vi "Manual.vi"(6 "Cluster":T12={"VISA resource name"="", "baud rate "=9600}, 7 "vi reference":refnum<vi>, 8 "error in (no error)":errorcluster, 9 "IOList_280":T1, 11 "Manual":T4(tab)) -> (0 "error out":errorcluster, 3 "Out reference":refnum<vi>)   [LabVIEW 2015]
uses:
  Control Button/Exit.ctl
  Control Button/Scanner config.ctl
  Control Button/Save.ctl
  Galobal variable_TI.vi
  <vilib>/addons/database/Connection.llb/DB Tools Open Connec (String).vi
  <vilib>/Instr/_visa.llb/VISA Configure Serial Port (Instr).vi
  <vilib>/addons/database/_DB Variant To Data/Database Variant To Data.xnode
  <vilib>/addons/database/NI_Database_API.lvlib
panel:
  out "Array":string[](array[string])
  out "Byte Lenth":i32
  out "error out 2":errorcluster
  out "Manual DO":bool[](array[boolean])
  in  "Stop":T2
  out "NewVal":T3
  in  "Digital Output":T5
  out "LVDT":string
  out "Digital Input":T6
  in  "Home Calling M1":bool
  in  "Stop M1":bool
  in  "SERVO ON CMD M1":bool
  in  "Speed (mm/s) M1":i32=10
  in  "Travel (mm)M1":i32=5
  out "STM1 Done Bit":bool
  out "Error Message":string
  out "Load Cell":dbl format="%0.03f"
  in  "Model Trigger":bool
  in  "Program List 2":string(combo)="VW Medium"
  out "Camera Status":T7
  in  "Save":T8
  out "Analog Input":T9 {"Analog Data 6" format="%0.02f"; "Analog Data 5" format="%0.02f"; "Analog Data 4" format="%0.02f"; "Analog Data 3" format="%0.02f"; "Analog Data 2" format="%0.02f"; "Analog Data" format="%0.02f"}
  in  "Sensor Data 3":T10
  out "Error Status":bool
  in  "Scanner config":T11
  out "Read data":string
  out "Boolean":bool
  # "Instruction for Servo motor Operate\n(1)  Switch  ON -OFF  of Fixture Slide servo Brake ON Cmd (P0.19)  \n      from Digital Output tab.\n(2) Switch  ON -OFF  of Fixture Slide Servo Direction Command (P0.20)\n      from Digital Output tab."
  # "Fixture Slide servo"
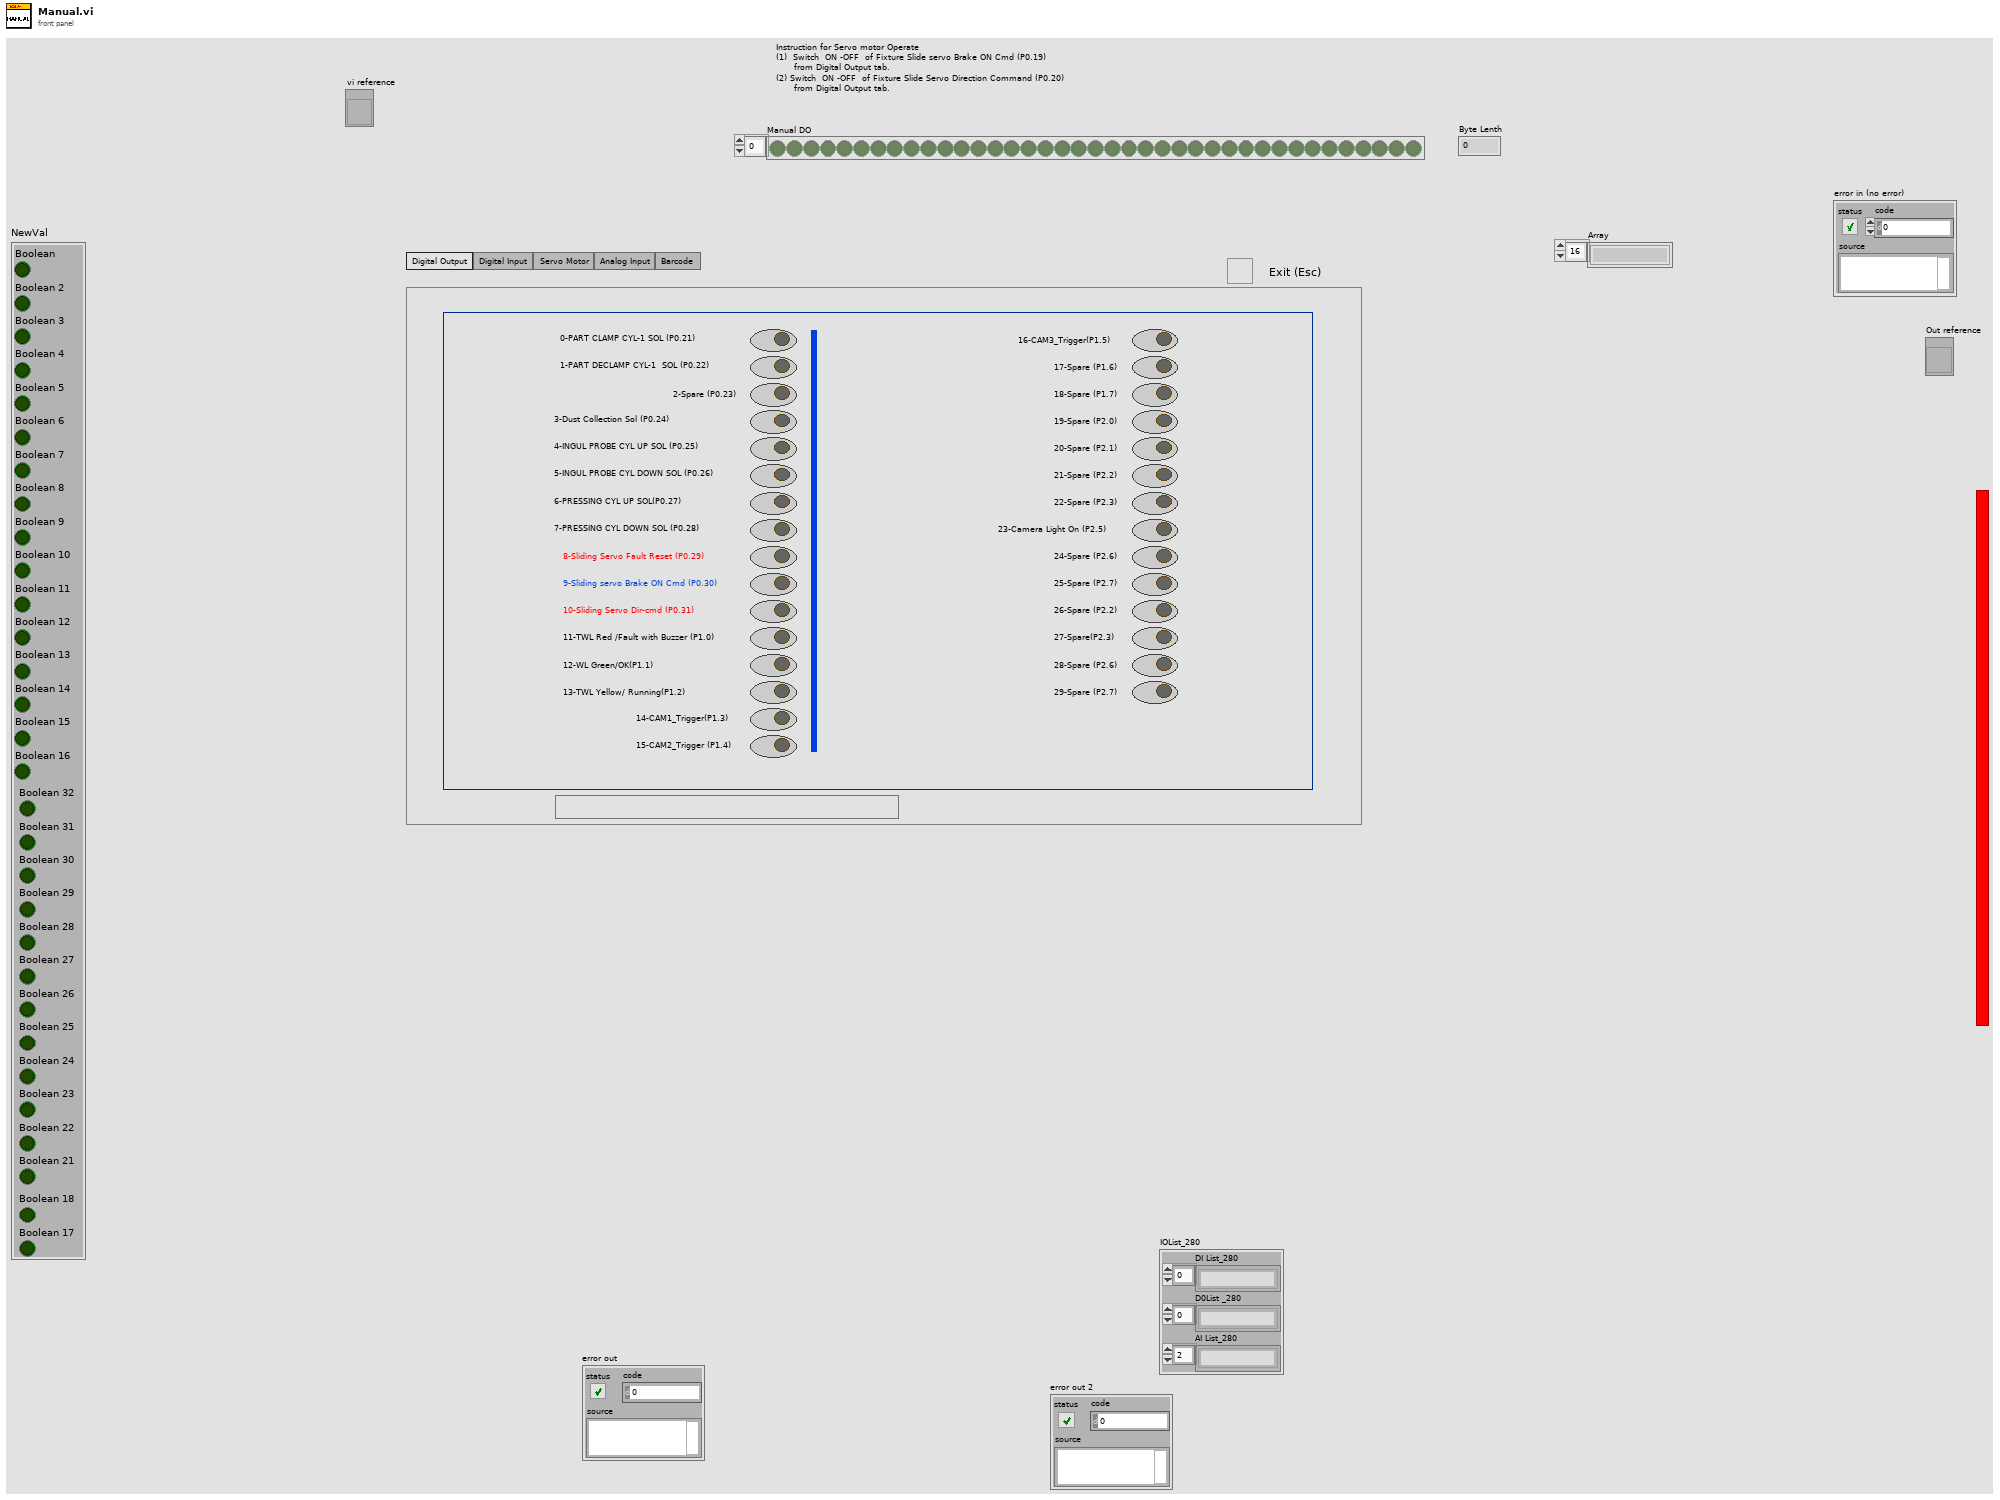
[diagram p1: front panel]
types:
  T1 = cluster{"DI List_280":string[], "D0List _280":string[], "AI List_280":string[]}
  T2 = typedef "Exit.ctl" = bool
  T3 = cluster{"Boolean":bool, "Boolean 2":bool, "Boolean 3":bool, "Boolean 4":bool, "Boolean 5":bool, "Boolean 6":bool, "Boolean 7":bool, "Boolean 8":bool, "Boolean 9":bool, "Boolean 10":bool, "Boolean 11":bool, "Boolean 12":bool, "Boolean 13":bool, "Boolean 14":bool, "Boolean 15":bool, "Boolean 16":bool, "Boolean 17":bool, "Boolean 18":bool, "Boolean 21":bool, "Boolean 22":bool, "Boolean 23":bool, "Boolean 24":bool, "Boolean 25":bool, "Boolean 26":bool, "Boolean 27":bool, "Boolean 28":bool, "Boolean 29":bool, "Boolean 30":bool, "Boolean 31":bool, "Boolean 32":bool}
  T4 = enum32{"Digital Output", "Digital Input", "Servo Motor ", "Analog Input", "Barcode "}
  T5 = cluster{"DO.00":bool, "DO.01":bool, "DO.02":bool, "DO.03":bool, "DO.04":bool, "DO.05":bool, "DO.06":bool, "DO.06":bool, "DO.07":bool, "DO.08":bool, "DO.09":bool, "DO.10":bool, "DO.11":bool, "DO.12":bool, "DO.13":bool, "DO.14":bool, "DO.07 2":bool, "DO.08 2":bool, "DO.09 2":bool, "DO.10 2":bool, "DO.11 2":bool, "DO.12 2":bool, "DO.13 2":bool, "DO.14 2":bool, "DO.00 2":bool, "DO.01 2":bool, "DO.02 2":bool, "DO.03 2":bool, "DO.06 2":bool, "DO.06 3":bool}
  T6 = cluster{"Digital Input":bool, "Digital Input 2":bool, "Digital Input 3":bool, "Digital Input 4":bool, "Digital Input 5":bool, "Digital Input 6":bool, "Digital Input 7":bool, "Digital Input 8":bool, "Digital Input 9":bool, "Digital Input 10":bool, "Digital Input 11":bool, "Digital Input 12":bool, "Digital Input 13":bool, "Digital Input 14":bool, "Digital Input 15":bool, "Digital Input 16":bool, "Digital Input 17":bool, "Digital Input 18":bool, "Digital Input 19":bool, "Digital Input 20":bool, "Digital Input 21":bool, "Digital Input 22":bool, "Digital Input 23":bool, "Digital Input 24":bool, "Digital Input 25":bool, "Digital Input 26":bool, "Digital Input 27":bool, "Digital Input 28":bool, "Digital Input 29":bool, "Digital Input 30":bool, "Digital Input 31":bool, "Digital Input 32":bool, "Digital Input 33":bool, "Digital Input 34":bool, "Digital Input 35":bool, "Digital Input 36":bool, "Digital Input 37":bool, "Digital Input 38":bool, "Digital Input 39":bool, "Digital Input 40":bool, "Digital Input 41":bool, "Digital Input 42":bool, "Digital Input 43":bool, "Digital Input 44":bool, "Digital Input 45":bool, "Digital Input 46":bool, "Digital Input 47":bool, "Digital Input 48":bool, "Digital Input 49":bool, "Digital Input 50":bool, "Digital Input 51":bool}
  T7 = cluster{"Left CAM OK":bool, "Left CAM NG":bool, "Right CAM OK":bool, "Right CAM NG":bool, "LCD  CAM OK":bool, "LCD CAM NG ":bool}
  T8 = typedef "Save.ctl" = bool
  T9 = cluster{"Analog Data":dbl, "Analog Data 2":dbl, "Analog Data 3":dbl, "Analog Data 4":dbl, "Analog Data 5":dbl, "Analog Data 6":dbl, "IL Sensor1_AI6":bool, "IL Sensor1_AI7":bool, "IL Sensor1_AI8":bool, "IL Sensor1_AI9":bool}
  T10 = cluster{"IL Sensor_Max (AI6)":dbl, "IL Sensor_Min (AI6)":dbl, "IL Sensor_Max (AI7)":dbl, "IL Sensor _Min (AI7)":dbl, "IL Sensor_Max (AI8)":dbl, "IL Sensor_Min (AI8)":dbl, "IL Sensor_Max  (AI9)":dbl, "IL Sensor_Min  (AI9)":dbl}
  T11 = typedef "Scanner config.ctl" = bool
  T12 = cluster{"VISA resource name":refnum<visa-resource-name>, "baud rate ":u32}
  T13 = typedef "NI_Database_API.lvlib/Conn ObjectReference.ctl" = refnum<k1>
  T14 = cluster{" Fixture Brack on":refnum<vi>, " Fixture Direction":refnum<vi>, "Servo Cmd":refnum<vi>, "Servo Home":refnum<vi>}
  T15 = cluster{"Digital input[0]":bool, "Digital input[1]":bool, "Digital input[2]":bool, "Digital input[3]":bool, "Digital input[4]":bool, "Digital input[5]":bool, "Digital input[6]":bool, "Digital input[7]":bool, "Digital input[8]":bool, "Digital input[9]":bool, "Digital input[10]":bool, "Digital input[11]":bool, "Digital input[12]":bool, "Digital input[13]":bool, "Digital input[14]":bool, "Digital input[15]":bool, "Digital input[16]":bool, "Digital input[17]":bool, "Digital input[18]":bool, "Digital input[19]":bool, "Digital input[20]":bool, "Digital input[21]":bool, "Digital input[22]":bool, "Digital input[23]":bool, "Digital input[24]":bool, "Digital input[25]":bool, "Digital input[26]":bool, "Digital input[27]":bool, "Digital input[28]":bool, "Digital input[29]":bool, "Digital input[30]":bool, "Digital input[31]":bool, "Digital input[32]":bool, "Digital input[33]":bool, "Digital input[34]":bool, "Digital input[35]":bool, "Digital input[36]":bool, "Digital input[37]":bool, "Digital input[38]":bool, "Digital input[39]":bool, "Digital input[40]":bool, "Digital input[41]":bool, "Digital input[42]":bool, "Digital input[43]":bool, "Digital input[44]":bool, "Digital input[45]":bool, "Digital input[46]":bool, "Digital input[47]":bool, "Digital input[48]":bool, "Digital input[49]":bool, "Digital input[50]":bool}
  T16 = cluster{"Load(AI0) ":dbl, "Load (AI1) ":dbl, "IL Sensor (AI6)":dbl, "IL Sensor  (AI7)":dbl, "IL Sensor (AI8)":dbl, "IL Sensor  (AI9)":dbl, "IL Sensor1_AI6":bool, "IL Sensor1_AI7":bool, "IL Sensor1_AI8":bool, "IL Sensor1_AI9":bool}
  T17 = cluster{"IL Sensor_Max (AI6)":dbl, "IL Sensor_Min (AI6)":dbl, "IL Sensor_Max (AI7)":dbl, "IL Sensor _Min (AI7)":dbl, "IL Sensor_Max (AI8)":dbl, "IL Sensor_Min (AI8)":dbl, "IL Sensor_Max  (AI9)":dbl, "IL Sensor_Min  (AI9)":dbl, "Key":string}
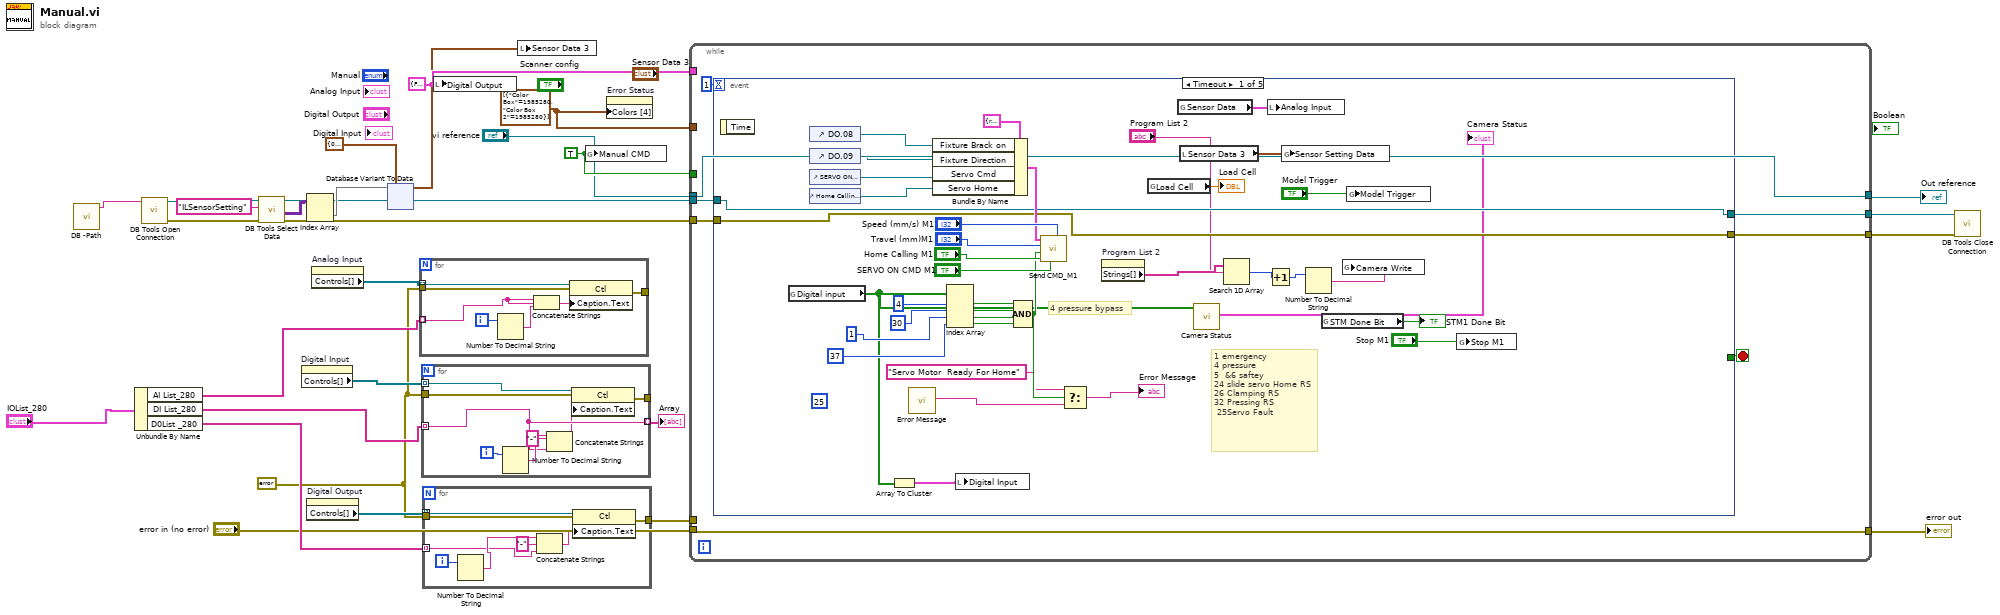
[diagram p0: block diagram]
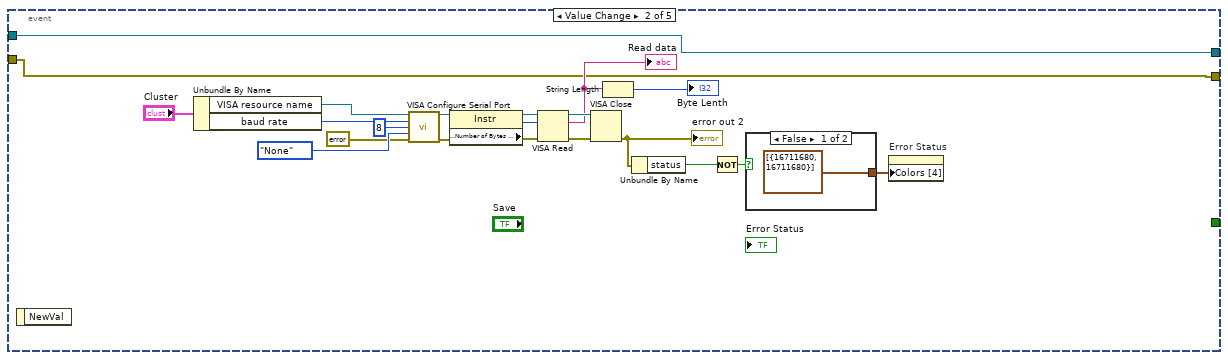
[diagram p2: hidden frame]
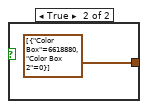
[diagram p3: hidden frame]
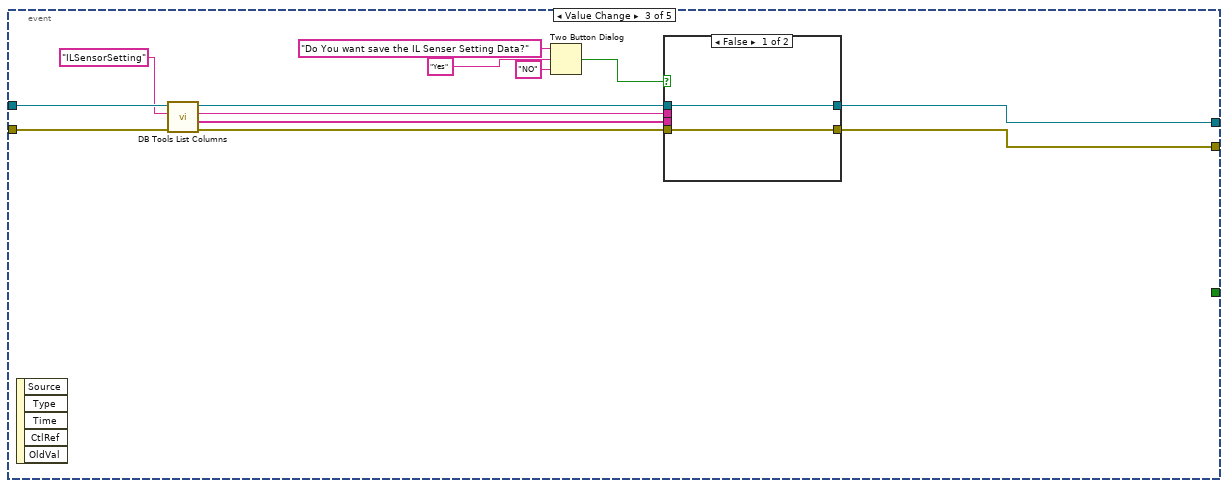
[diagram p4: hidden frame]
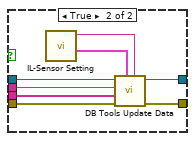
[diagram p5: hidden frame]
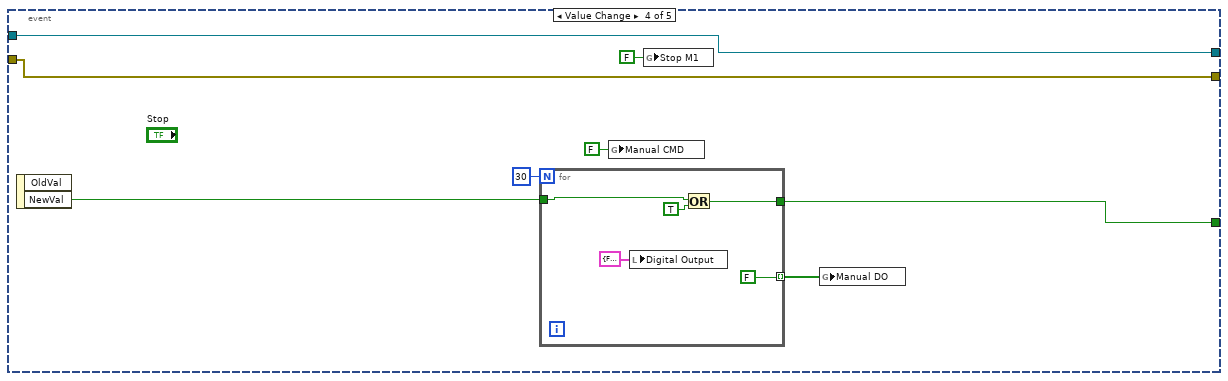
[diagram p6: hidden frame]
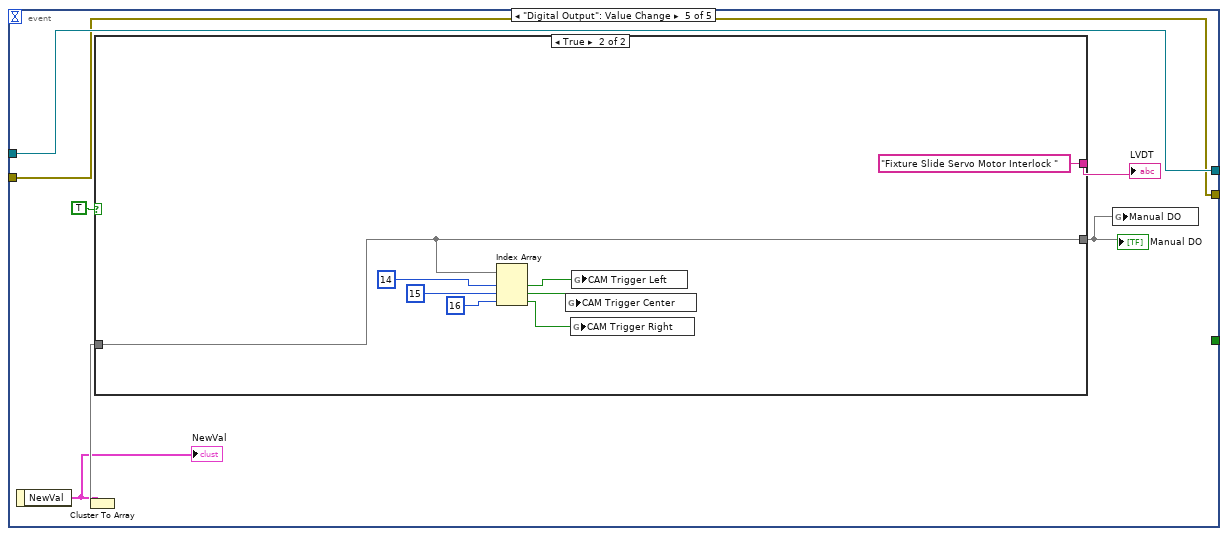
[diagram p7: hidden frame]
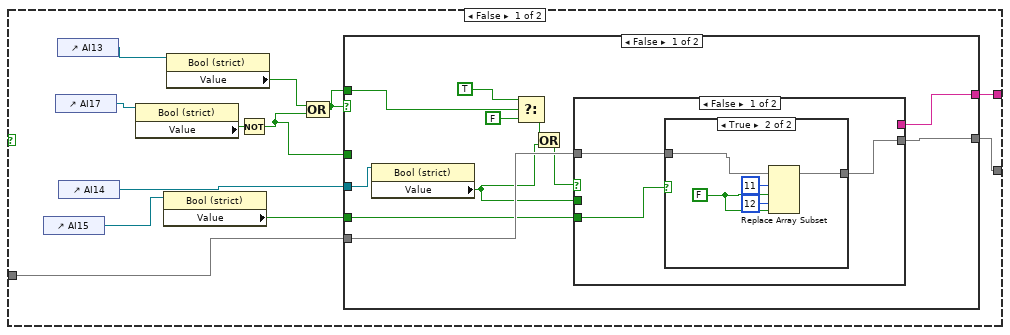
[diagram p8: hidden frame]
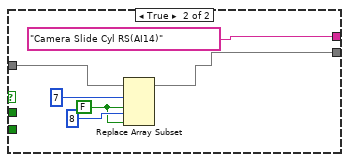
[diagram p10: hidden frame]
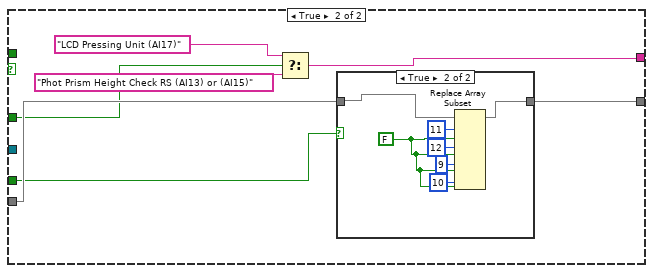
[diagram p11: hidden frame]
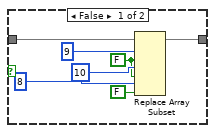
[diagram p12: hidden frame]
diagram:
  w13 = T5 {"DO.00"=FALSE, "DO.01"=FALSE, "DO.02"=FALSE, "DO.03"=FALSE, "DO.04"=FALSE, "DO.05"=FALSE, "DO.06"=FALSE, "DO.06"=FALSE, "DO.07"=FALSE, "DO.08"=FALSE, "DO.09"=FALSE, "DO.10"=FALSE, "DO.11"=FALSE, "DO.12"=FALSE, "DO.13"=FALSE, "DO.14"=FALSE, "DO.07 2"=FALSE, "DO.08 2"=FALSE, "DO.09 2"=FALSE, "DO.10 2"=FALSE, "DO.11 2"=FALSE, "DO.12 2"=FALSE, "DO.13 2"=FALSE, "DO.14 2"=FALSE, "DO.00 2"=FALSE, "DO.01 2"=FALSE, "DO.02 2"=FALSE, "DO.03 2"=FALSE, "DO.06 2"=FALSE, "DO.06 3"=FALSE} ("Digital Output")
  w16 = errorcluster {"status"=FALSE, "code"=0, "source"=""} ("error in (no error)")
  w19 = cluster{"Color Box":u32, "Color Box 2":u32}[] [{"Color Box"=1985280, "Color Box 2"=1985280}] ("Colors [4]")
  w25 = TRUE ("Manual CMD")
  n1 = call "DB -Path.vi"() -> ("String"=w8:string)  [unwired: 11 in]
  n2 = Unbundle By Name("IOList_280") -> ("AI List_280"=w20:string[], "DI List_280"=w22:string[], "D0List _280"=w24:string[])
  n3 = call-poly <vilib>:"DB Tools Open Connection.vi"("connection information"=w8) -> ("error out"=w6:errorcluster, "connection reference"=w7:T13)  [unwired: 7 in]
  n4 = call <vilib>:"DB Tools Select Data.vi"("error in (no error)"=w6, "table"="ILSensorSetting", "connection reference"=w7) -> ("error out"=w4:errorcluster, "data"=w9:variant[][], "connection reference out"=w5:T13)  [unwired: 3 in]
  n5 = property on="Digital Input" class="Clust (strict)"() -> ("Controls[]"=w23:refnum<vi>[])  [unwired: 2 in, 2 out]
  n6 = Index Array(array=w9) -> (element=w10:variant[])  [unwired: 2 in]
  n7 = property on="Digital Output" class="Clust (strict)"() -> ("Controls[]"=w28:refnum<vi>[])  [unwired: 2 in, 2 out]
  n8 = property on="Analog Input" class="Clust (strict)"() -> ("Controls[]"=w21:refnum<vi>[])  [unwired: 2 in, 2 out]
  n9 = xnode "Database Variant To Data"("database variant"=w10, "type"=T10 {"IL Sensor_Max (AI6)"=0.0, "IL Sensor_Min (AI6)"=0.0, "IL Sensor_Max (AI7)"=0.0, "IL Sensor _Min (AI7)"=0.0, "IL Sensor_Max (AI8)"=0.0, "IL Sensor_Min (AI8)"=0.0, "IL Sensor_Max  (AI9)"=0.0, "IL Sensor_Min  (AI9)"=0.0} ("Sensor Setting Data")) -> ("data"=w1:T10)  [unwired: 1 in, 1 out]
  n10 = for {
    tunnel: w21 -> [w35] mode=indexing
    tunnel: [w33] -> _
    tunnel: w16 -> [w31]
    tunnel: w20 -> [w30] mode=indexing
    i -> [w34]
    n11 = Number To Decimal String(number=w34) -> (decimal integer string=w32:string)  [unwired: 1 in]
    n12 = Concatenate Strings(w30, w32) -> ()  [unwired: 1 out]
    n13 = property class="Ctl"(reference=w35, error in=w31, "Caption.Text"=w30) -> (error out=w33:errorcluster)  [unwired: 1 out]
  }
  n14 = for {
    tunnel: w23 -> [w43] mode=indexing
    tunnel: [w41] -> _
    tunnel: w16 -> [w40]
    tunnel: w22 -> [w37] mode=indexing
    tunnel: [w37] -> w17 mode=indexing
    i -> [w42]
    n15 = Number To Decimal String(number=w42) -> (decimal integer string=w39:string)  [unwired: 1 in]
    n16 = Concatenate Strings(w39, "-" ("string"), w37) -> (w36:string)
    n17 = property class="Ctl"(reference=w43, error in=w40, "Caption.Text"=w36) -> (error out=w41:errorcluster)  [unwired: 1 out]
  }
  "Array" <- w17
  n18 = for {
    tunnel: w28 -> [w51] mode=indexing
    tunnel: [w49] -> w29
    tunnel: w16 -> [w48]
    tunnel: w24 -> [w44] mode=indexing
    i -> [w50]
    n19 = Number To Decimal String(number=w50) -> (decimal integer string=w45:string)  [unwired: 1 in]
    n20 = Concatenate Strings(w45, "-" ("string"), w44) -> (w47:string)
    n21 = property class="Ctl"(reference=w51, error in=w48, "Caption.Text"=w47) -> (error out=w49:errorcluster)  [unwired: 1 out]
  }
  n22 = local write "Digital Output"(w13) -> ()
  n23 = local write "Sensor Data 3"(w1) -> ()
  n24 = global write "Galobal variable_TI.vi" "Manual CMD"(w25) -> ()
  n25 = property on="Error Status" class="Bool (strict)"("Colors [4]"=w19) -> ()  [unwired: 2 in, 2 out]
  n26 = while {
    tunnel: w29 -> [_]
    tunnel: [w57] -> w27
    tunnel: "vi reference" -> [w58]
    tunnel: [w58] -> w26
    tunnel: w25 -> [_]
    tunnel: w19 -> [_]
    tunnel: "error in (no error)" -> [w57]
    tunnel: w13 -> [_]
    tunnel: w5 -> [w55]
    tunnel: w4 -> [w54]
    tunnel: [w53] -> w3
    tunnel: [w52] -> w2
    stop <- w56 stop-if-true
    n27 = event shown="[0] Timeout" {
      selector: _ -> [_ _ _ _ _]
      dyn-events: _ -> [_ _ _ _ _]
      timeout: 1 -> [_ _ _ _ _]
      tunnel: [_ _ _ w145 _] -> w56
      tunnel: w55 -> [w71 w99 w132 w144 w157]
      tunnel: w54 -> [w70 w98 w131 w143 w156]
      tunnel: [w71 w99 w126 w144 w157] -> w53
      tunnel: [w70 w98 w125 w143 w156] -> w52
      event Timeout {
        (unwired) 25 ("index")
        # "4 pressure bypass"
        # "1 emergency\n4 pressure\n5  &6 saftey\n24 slide servo Home RS\n26 Clamping RS\n32 Pressing RS \n 25Servo Fault"
        n28 = event-data() -> ()  [unwired: 1 in, 1 out]
        n29 = global read "Galobal variable_TI.vi" "Digital input"() -> (w61:bool[])
        n30 = control-ref of="DO.08"() -> (w75:refnum<vi>)
        n31 = control-ref of="DO.09"() -> (w74:refnum<vi>)
        n32 = control-ref of="SERVO ON CMD M1"() -> (w89:refnum<vi>)
        n33 = control-ref of="Home Calling M1"() -> (w90:refnum<vi>)
        n34 = Array To Cluster(array=w61) -> (cluster=w97:T15)
        n35 = call "Error Message.vi"() -> ("Error"=w80:string)  [unwired: 11 in]
        n36 = Bundle By Name(cluster=T14 {" Fixture Brack on"=refnum, " Fixture Direction"=refnum, "Servo Cmd"=refnum, "Servo Home"=refnum} ("Slide Servo"), "Fixture Brack on"=w75, "Fixture Direction"=w74, "Servo Cmd"=w89, "Servo Home"=w90) -> (w88:T14)
        n37 = Index Array(array=w61, index #1=4 ("index"), index #2=30 ("index"), index #3=1 ("index"), index #4=37 ("index")) -> (element #1=w84:bool, element #2=w76:bool, element #3=w69:bool, element #4=w78:bool)
        n38 = local write "Digital Input"(w97) -> ()
        n39 = Compound Arithmetic op=AND(w84, w76, w69, w78) -> (w82:bool)
        n40 = call "Send CMD_M1.vi"("Speed (mm/s) M1"="Speed (mm/s) M1", "SERVO ON CMD M1"="SERVO ON CMD M1", "Home Calling M1"="Home Calling M1", "Pokayoka"=w82, "Travel (mm)M1"="Travel (mm)M1", "Slide Servo"=w88) -> ()  [unwired: 6 in]
        n41 = Select(t="Servo Motor  Ready For Home", s=w82, f=w80) -> (s? t:f=→"Error Message":string)
        n42 = property on="Program List 2" class="CmbBox"() -> ("Strings[]"=w63:string[])  [unwired: 2 in, 2 out]
        n43 = global read "Galobal variable_TI.vi" "Load Cell"() -> (→"Load Cell":dbl)
        n44 = global read "Galobal variable_TI.vi" "Sensor Data"() -> (w73:T16)
        n45 = local read "Sensor Data 3"() -> (w72:T10)
        n46 = call "Camera Status.vi"("Digital input"=w61) -> ("Camera Status"=→"Camera Status":T7)  [unwired: 10 in]
        n47 = Search 1D Array(1D array=w63, element="Program List 2") -> (index of element=w65:i32)  [unwired: 1 in]
        n48 = local write "Analog Input"(w73) -> ()
        n49 = Increment(x=w65) -> (x+1=w66:i32)
        n50 = global write "Galobal variable_TI.vi" "Sensor Setting Data"(w72) -> ()
        n51 = Number To Decimal String(number=w66) -> (decimal integer string=w67:string)  [unwired: 1 in]
        n52 = global read "Galobal variable_TI.vi" "STM Done Bit"() -> (→"STM1 Done Bit":bool)
        n53 = global write "Galobal variable_TI.vi" "Camera Write"(w67) -> ()
        n54 = global write "Galobal variable_TI.vi" "Model Trigger"("Model Trigger") -> ()
        n55 = global write "Galobal variable_TI.vi" "Stop M1"("Stop M1") -> ()
      }
      event Value Change {
        n56 = event-data() -> ()  [unwired: 1 in, 1 out]
        n57 = Unbundle By Name("Cluster") -> ("VISA resource name"=w118:refnum<visa-resource-name>, "baud rate"=w117:u32)
        n58 = call-poly "VISA Configure Serial Port"("VISA resource name"=w118, "baud rate (9600)"=w117, "data bits (8)"=u16 8, "parity (0:none)"=enum16{"None", "Odd", "Even", "Mark", "Space"}."None", "error in (no error)"=errorcluster {"status"=FALSE, "code"=0, "source"=""} ("error in (no error) 2")) -> ("VISA resource name out"=w116:refnum<visa-resource-name>, "error out"=w114:errorcluster)  [unwired: 9 in]
        n59 = property class="Instr"(reference=w116, error in=w114) -> (reference out=w115:refnum<visa-resource-name>, error out=w113:errorcluster, "Serial Settings:Number of Bytes at Serial Port"=w112:u32)
        n60 = VISA Read(VISA resource name=w115, byte count=w112, error in (no error)=w113) -> (VISA resource name out=w110:refnum<visa-resource-name>, read buffer=w108:string, error out=w109:errorcluster)  [unwired: 1 out]
        "Read data" <- w108
        n61 = VISA Close(VISA resource name=w110, error in (no error)=w109) -> (error out=w106:errorcluster)
        "error out 2" <- w106
        n62 = String Length(string=w108) -> (length=→"Byte Lenth":i32)
        n63 = Unbundle By Name(w106) -> ("status"=w105:bool)
        n64 = Not(x=w105) -> (.not. x?=w103:bool)
        n65 = case shown="False" w103 {
          tunnel: [cluster{"Color Box":u32, "Color Box 2":u32}[] [{"Color Box"=16711680, "Color Box 2"=16711680}] ("Colors [4]") cluster{"Color Box":u32, "Color Box 2":u32}[] [{"Color Box"=6618880, "Color Box 2"=0}] ("Colors [4]")] -> w104
          frame False {
          }
          frame True {
          }
        }
        n66 = property on="Error Status" class="Bool (strict)"("Colors [4]"=w104) -> ()  [unwired: 2 in, 2 out]
      }
      event Value Change {
        w128 = "ILSensorSetting" ("table")
        n67 = event-data() -> ()  [unwired: 1 in, 5 out]
        n68 = call <vilib>:"DB Tools List Columns.vi"("error in (no error)"=w131, "table"=w128, "connection reference"=w132) -> ("error out"=w129:errorcluster, "columns"=w127:string[], "connection reference out"=w130:T13)  [unwired: 1 in, 1 out]
        n69 = Two Button Dialog(message="Do You want save the IL Senser Setting Data?", 1:"NO" ("F button name (\"Cancel\")"), 2:"Yes" ("T button name (\"OK\")")) -> (T button?=w124:bool)
        n70 = case shown="False" w124 {
          tunnel: w130 -> [w134 w142]
          tunnel: w129 -> [w133 w141]
          tunnel: w128 -> [_ w140]
          tunnel: w127 -> [_ w139]
          tunnel: [w134 w136] -> w126
          tunnel: [w133 w135] -> w125
          frame False {
          }
          frame True {
            n71 = call "IL-Sensor Setting.vi"() -> ("IL Sensor"=w137:T17, "Search Key"=w138:string)  [unwired: 10 in]
            n72 = call <vilib>:"DB Tools Update Data.vi"("condition"=w138, "data"=w137, "error in (no error)"=w141, "columns"=w139, "table"=w140, "connection reference"=w142) -> ("error out"=w135:errorcluster, "connection reference out"=w136:T13)  [unwired: 4 in]
          }
        }
      }
      event Value Change {
        n73 = event-data() -> ("NewVal"=w146:T2)  [unwired: 1 in, 1 out]
        n74 = for {
          N: 30 -> [_]
          tunnel: [FALSE] -> w148 mode=indexing
          tunnel: w146 -> [w153]
          tunnel: [w152] -> w145
          n75 = local write "Digital Output"(T5 {"DO.00"=FALSE, "DO.01"=FALSE, "DO.02"=FALSE, "DO.03"=FALSE, "DO.04"=FALSE, "DO.05"=FALSE, "DO.06"=FALSE, "DO.06"=FALSE, "DO.07"=FALSE, "DO.08"=FALSE, "DO.09"=FALSE, "DO.10"=FALSE, "DO.11"=FALSE, "DO.12"=FALSE, "DO.13"=FALSE, "DO.14"=FALSE, "DO.07 2"=FALSE, "DO.08 2"=FALSE, "DO.09 2"=FALSE, "DO.10 2"=FALSE, "DO.11 2"=FALSE, "DO.12 2"=FALSE, "DO.13 2"=FALSE, "DO.14 2"=FALSE, "DO.00 2"=FALSE, "DO.01 2"=FALSE, "DO.02 2"=FALSE, "DO.03 2"=FALSE, "DO.06 2"=FALSE, "DO.06 3"=FALSE} ("Digital Output")) -> ()
          n76 = Or(x=w153, y=TRUE) -> (x .or. y?=w152:T2)
        }
        n77 = global write "Galobal variable_TI.vi" "Manual CMD"(FALSE ("Manual CMD")) -> ()
        n78 = global write "Galobal variable_TI.vi" "Stop M1"(FALSE ("Stop M1")) -> ()
        n79 = global write "Galobal variable_TI.vi" "Manual DO"(w148) -> ()
      }
      event "Digital Output": Value Change {
        n80 = event-data() -> ("NewVal"=w158:T5)  [unwired: 1 in]
        "NewVal" <- w158
        n81 = Cluster To Array(cluster=w158) -> (array=w159:bool[])
        n82 = case shown="True" TRUE ("By Pass") {
          tunnel: [w173 w228] -> w162
          tunnel: [w171 "Fixture Slide Servo Motor Interlock "] -> w161
          tunnel: w159 -> [w164 w228]
          frame False {
            n83 = control-ref of="AI15"() -> (w165:refnum<vi>)
            n84 = control-ref of="AI17"() -> (w168:refnum<vi>)
            n85 = control-ref of="AI13"() -> (w172:refnum<vi>)
            n86 = control-ref of="AI14"() -> (w174:refnum<vi>)
            n87 = property class="Bool (strict)"(reference=w168) -> ("Value"=w169:bool)  [unwired: 1 in, 2 out]
            n88 = property class="Bool (strict)"(reference=w165) -> ("Value"=w163:bool)  [unwired: 1 in, 2 out]
            n89 = property class="Bool (strict)"(reference=w172) -> ("Value"=w170:bool)  [unwired: 1 in, 2 out]
            n90 = Not(x=w169) -> (.not. x?=w167:bool)
            n91 = Compound Arithmetic op=OR(w170, w167) -> (w166:bool)
            n92 = case shown="False" w166 {
              tunnel: w164 -> [w185 w207]
              tunnel: w174 -> [w184 _]
              tunnel: [w183 w206] -> w173
              tunnel: [w182 w202] -> w171
              tunnel: w167 -> [_ w205]
              tunnel: w166 -> [w181 _]
              tunnel: w163 -> [w175 w201]
              frame False {
                n93 = property class="Bool (strict)"(reference=w184) -> ("Value"=w177:bool)  [unwired: 1 in, 2 out]
                n94 = Select(t=TRUE, s=w181, f=FALSE) -> (s? t:f=w178:bool)
                n95 = Or(x=w178, y=w177) -> (x .or. y?=w176:bool)
                n96 = case shown="False" w176 {
                  tunnel: w185 -> [w187 w198]
                  tunnel: [w186 w197] -> w183
                  tunnel: w177 -> [_ _]
                  tunnel: [_ "Camera Slide Cyl RS(AI14)"] -> w182
                  tunnel: w175 -> [w188 _]
                  frame False {
                    n97 = case shown="True" w188 {
                      tunnel: w187 -> [w189 w192]
                      tunnel: [w189 w191] -> w186
                      frame False {
                      }
                      frame True {
                        w190 = FALSE ("new element/subarray")
                        n98 = Replace Array Subset(array=w192, new element #1=w190, index #1=11 ("index"), new element #2=w190, index #2=12 ("index")) -> (w191:bool[])
                      }
                    }
                  }
                  frame True {
                    w195 = FALSE ("new element/subarray")
                    n99 = Replace Array Subset(array=w198, new element #1=w195, index #1=7 ("index"), new element #2=w195, index #2=8 ("index")) -> (w197:bool[])
                  }
                }
              }
              frame True {
                n100 = Select(t="LCD Pressing Unit (AI17)", s=w205, f="Phot Prism Height Check RS (AI13) or (AI15)") -> (s? t:f=w202:string)
                n101 = case shown="True" w201 {
                  tunnel: w207 -> [w211 w219]
                  tunnel: [w210 w218] -> w206
                  frame False {
                    w212 = FALSE ("new element/subarray")
                    n102 = Replace Array Subset(array=w211, new element #1=w212, index #1=9 ("index"), new element #2=w212, index #2=10 ("index"), new element #3=FALSE ("new element/subarray"), index #3=8 ("index")) -> (w210:bool[])
                  }
                  frame True {
                    w215 = FALSE ("new element/subarray")
                    n103 = Replace Array Subset(array=w219, new element #1=w215, index #1=11 ("index"), new element #2=w215, index #2=12 ("index"), new element #3=w215, index #3=9 ("index"), new element #4=w215, index #4=10 ("index")) -> (w218:bool[])
                  }
                }
              }
            }
          }
          frame True {
            n104 = Index Array(array=w228, index #1=14 ("index"), index #2=15 ("index"), index #3=16 ("index")) -> (element #1=w224:bool, element #2=w223:bool, element #3=w222:bool)
            n105 = global write "Galobal variable_TI.vi" "CAM Trigger Center"(w223) -> ()
            n106 = global write "Galobal variable_TI.vi" "CAM Trigger Right"(w222) -> ()
            n107 = global write "Galobal variable_TI.vi" "CAM Trigger Left"(w224) -> ()
          }
        }
        "Manual DO" <- w162
        "LVDT" <- w161
        n108 = global write "Galobal variable_TI.vi" "Manual DO"(w162) -> ()
      }
    }
  }
  "error out" <- w27
  "Out reference" <- w26
  n109 = call <vilib>:"DB Tools Close Connection.vi"("error in (no error)"=w2, "connection reference"=w3) -> ()  [unwired: 5 in, 1 out]
